vi "MSEncoder SubVI EndofProcess.vi"(8 "error in (no error)":errorcluster, 11 "MSEncoder in":refnum<class "MSEncoder.lvclass">) -> (0 "error out":errorcluster, 3 "MS Encoder":refnum<class "MSEncoder.lvclass">)   [LabVIEW 2018, in "MSEncoder.lvclass"]
uses:
  MSEncoder.lvclass
  PublicSubVI/Class/SigInfo/SigInfo.ctl
  MSEncoder.lvclass/MSEncoder.ctl
  PublicSubVI/Class/SigInfo/SigInfo.lvclass
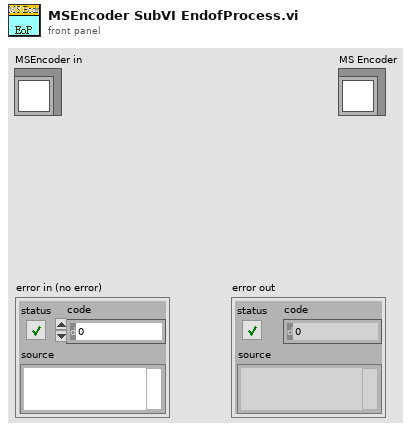
[diagram p1: front panel]
types:
  T1 = typedef "SigInfo.ctl" = enum16{"New mzList", "Set SigInfo", "Get SigInfo", "Append", "End"}
  T2 = cluster{"Label":string, "dt":dbl, "Length":u32, "RefVolt":dbl, "mzTable":cluster{"t":dbl[], "mz":dbl[], "beta":dbl[]}}[]
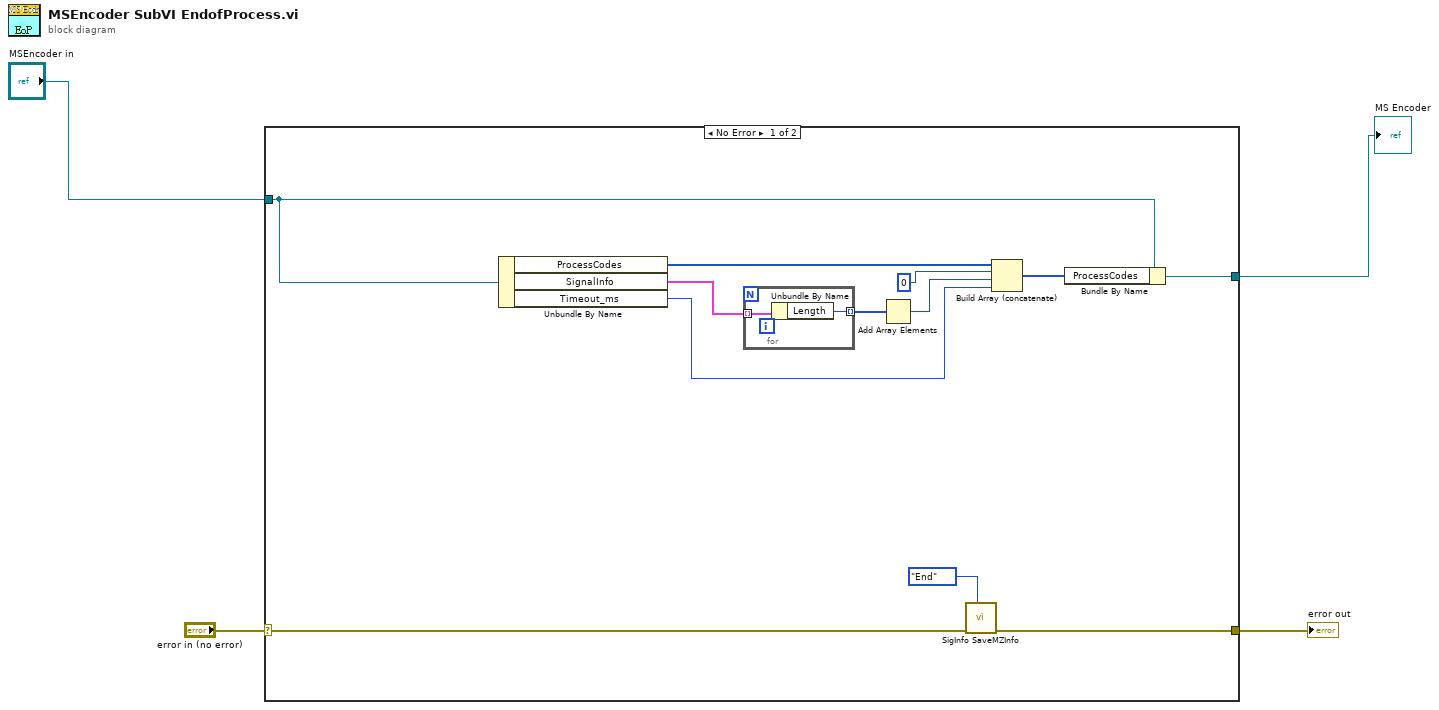
[diagram p0: block diagram]
diagram:
  n1 = case shown="No Error" "error in (no error)" {
    selector: "error in (no error)" -> [w7 w20]
    tunnel: [w6 w20] -> w3
    tunnel: "MSEncoder in" -> [w5 w19]
    tunnel: [w10 w19] -> w1
    frame No Error {
      n2 = Unbundle By Name(w5) -> ("ProcessCodes"=w15:u64[], "SignalInfo"=w14:T2, "Timeout_ms"=w9:i32)
      n3 = for {
        tunnel: w14 -> [w18] mode=indexing
        tunnel: [w17] -> w13 mode=indexing
        n4 = Unbundle By Name(w18) -> ("Length"=w17:u32)
      }
      n5 = Add Array Elements(numeric array=w13) -> (sum=w12:u32)
      n6 = call "SigInfo SaveMZInfo.vi"("Function"=SigInfo."End", "error in (no error)"=w7) -> ("error out"=w6:errorcluster)  [unwired: 7 in, 2 out]
      n7 = Build Array (concatenate)(w15, u64 0, w12, w9) -> (w11:u64[])
      n8 = Bundle By Name(cluster=w5, "ProcessCodes"=w11) -> (w10:refnum<class "MSEncoder.lvclass">)
    }
    frame Error {
    }
  }
  "error out" <- w3
  "MS Encoder" <- w1
